vi "cmd Stop.vi"(8 "error in (no error)":errorcluster, 11 "IUI_Command in":refnum<class "IUI_Command.lvclass">) -> (0 "error out":errorcluster, 3 "IUI_Command out":refnum<class "IUI_Command.lvclass">)   [LabVIEW 2020, in "Main_UI.lvlib" / "IUI_Command.lvclass"]
uses:
  IUI_Command.lvclass
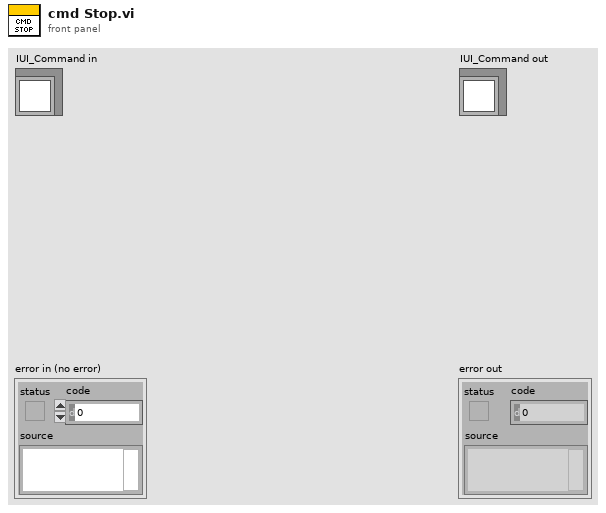
[diagram p1: front panel]
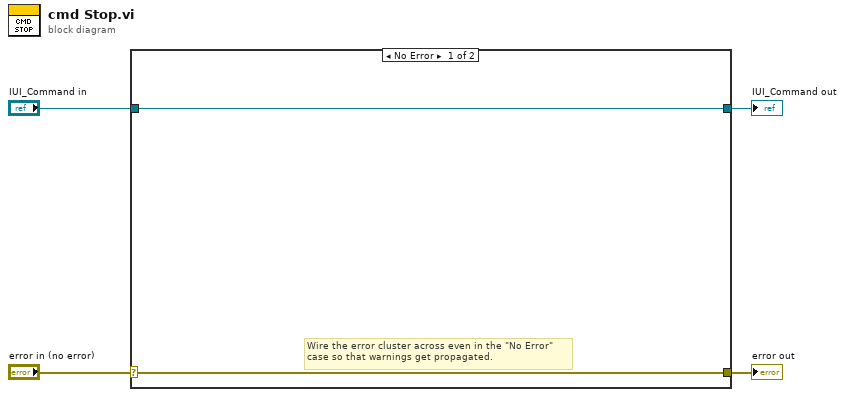
[diagram p0: block diagram]
diagram:
  n1 = case shown="No Error" "error in (no error)" {
    selector: "error in (no error)" -> [w5 w8]
    tunnel: [w5 w8] -> w3
    tunnel: [w6 w7] -> w1
    tunnel: "IUI_Command in" -> [w6 w7]
    frame No Error {
      # "Wire the error cluster across even in the \"No Error\"\ncase so that warnings get propagated."
    }
    frame Error {
    }
  }
  "error out" <- w3
  "IUI_Command out" <- w1
